vi "Copy C Image To Lab VIEW Image.vi"(7 "LVHeight":i32, 8 "error in (no error)":errorcluster, 9 "LVWidth":i32, 10 "LVLineWidth":i32, 11 "LVImagePtr":string) -> (0 "error out":errorcluster, 2 "function return":i32, 3 "LVImagePtr out":string)   [LabVIEW 2017, in "BonTechWrapperLibrary.lvlib"]
doc: "extern \"C\" BONTECHLIBRARY_API int __stdcall Copy_C_Image_To_LabVIEW_Image(char* LVImagePtr, int LVLineWidth, int LVWidth, int LVHeight);"
uses:
  BonTechWrapperLibrary.lvlib
  BonTechWrapperLibrary.dll
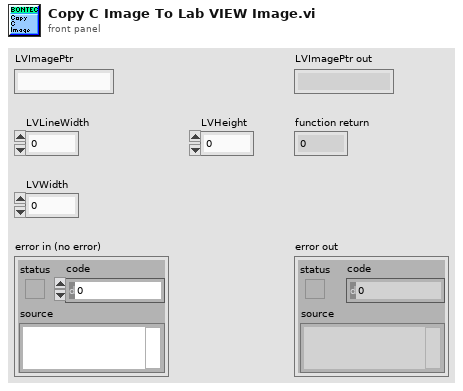
[diagram p1: front panel]
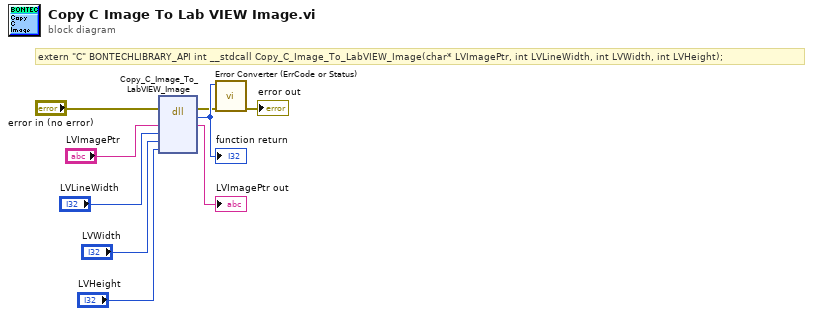
[diagram p0: block diagram]
diagram:
  # "extern \"C\" BONTECHLIBRARY_API int __stdcall Copy_C_Image_To_LabVIEW_Image(char* LVImagePtr, int LVLineWidth, int LVWidth, int LVHeight);"
  n1 = dll-call lib="C:/Users/Achuthaperumal/SourceCodes/BonTechWrapperLibrary/BonTechWrapperLibrary/x64/Release/BonTechWrapperLibrary.*" fn="Copy_C_Image_To_LabVIEW_Image"(error in="error in (no error)", "LVImagePtr"="LVImagePtr", "LVLineWidth"="LVLineWidth", "LVWidth"="LVWidth", "LVHeight"="LVHeight") -> (error out=w2:errorcluster, w9:i32, "LVImagePtr"=→"LVImagePtr out":string)  [unwired: 5 in, 1 out]
  "function return" <- w9
  n2 = call "Error Converter (ErrCode or Status).vi"("error in (no error)"=w2, "error code"=w9) -> ("error out"=→"error out":errorcluster)  [unwired: 9 in]
